vi "Restart.CheckValidSelection.vi"(8 "error in (no error)":errorcluster, 10 "Restart Path":path, 11 "State Variables":T1={"Events.State"=refnum, "Events.Test Result"=refnum, "Events.Progress"=refnum, "INI.Settings"={"Build Location"=path "C:/Simple Sequence Editor/SequenceRepo", "LoggingLocation"=path "", "Sequence.AbortChannel"="", "Sequence.IterationInfoChannel"="", "Sequence.DurationChannel"="", "Sequence.StepInfoChannel"="", "Sequence.SkipChannel"="", "PlotChannels"=[], "Sequence.InitializeScript"=path "C:/Simple Sequence Editor/SequenceRepo", "Sequence.CleanupScript"=path "", "Log.DefaultRate"=0.0}, "NIVS.AlarmManager"=refnum, "NIVS.BaseLogPath"=path "", "NIVS.DataLogManagerRef"=refnum, "NIVS.DataLogSpecRef"=refnum, "NIVS.Deployed"=FALSE, "NIVS.Events"={"SequenceEvent"=refnum, "SystemChangeEvent"=refnum, "WorkspaceEvent"=refnum}, "NIVS.GatewayIPAddress"="", "NIVS.DataLogGUID"="", "NIVS.ProfileCallback"=refnum, "NIVS.ProfileRef"=refnum, "NIVS.SequenceState"=enum."Idle", "NIVS.SystemDefinitionFile"=path "", "NIVS.SystemStateRefs"={"CustDatRef"=refnum, "EvtRef"=refnum, "Target State User Event"=refnum}, "NIVS.WorkspaceManager"=refnum, "NIVS.EventLogGUID"="", "NIVS.EventLogManagerRef"=refnum, "NIVS.EventLogSpecRef"=refnum, "NIVS.BaseToolPath"=path "", "Restart.Path"=path "", "Sequence.#ofColumns"=0, "Sequence.Iterations"=0, "Sequence.Channels"=[], "Sequence.ValidConfig?"=FALSE, "Station.ID"="", "UDP.Queue"=refnum, "UI.Abort"=refnum, "UI.Alarms"=refnum, "UI.Apply"=refnum, "UI.Back"=refnum, "UI.BaseFileName"=refnum, "UI.CurrentIteration"=refnum, "UI.CurrentStep"=refnum, "UI.CyclicFrequency"=refnum, "UI.Description"=refnum, "UI.DelayTime"=refnum, "UI.DisableAlarms"=refnum, "UI.Duration"=refnum, "UI.EnableLogging"=refnum, "UI.EnableState"=refnum, "UI.High"=refnum, "UI.LogChannels"=refnum, "UI.Low"=refnum, "UI.MonitoredVariable"=refnum, "UI.Next"=refnum, "UI.NumberOfCycles"=refnum, "UI.OperatorName"=refnum, "UI.Pause"=refnum, "UI.Profile"=refnum, "UI.Revert"=refnum, "UI.Skip"=refnum, "UI.Start"=refnum, "UI.StartIteration"=refnum, "UI.StartStep"=refnum, "UI.TabControl"=refnum, "UI.TotalIterations"=refnum, "UI.WaveformDefinition"=refnum, "UI.WaveformPreview"=refnum, "UI.WorkOrderNumber"=refnum, "UI.Chart"=refnum, "UI.Status"=refnum, "UI.DataView"=refnum, "UI.Table"=refnum, "UI.Multihead"=refnum, "UI.ToolTab"=refnum, "UI.Result"=refnum, "UI.Log Path"=refnum, "UI.ReportPath"=refnum, "UI.RestartPath"=refnum, "UI.AlarmLog"=refnum}) -> (0 "error out":errorcluster, 2 "Load Restart?":bool, 3 "State Variables out":T1={"Events.State"=refnum, "Events.Test Result"=refnum, "Events.Progress"=refnum, "INI.Settings"={"Build Location"=path "C:/Simple Sequence Editor/SequenceRepo", "LoggingLocation"=path "", "Sequence.AbortChannel"="", "Sequence.IterationInfoChannel"="", "Sequence.DurationChannel"="", "Sequence.StepInfoChannel"="", "Sequence.SkipChannel"="", "PlotChannels"=[], "Sequence.InitializeScript"=path "C:/Simple Sequence Editor/SequenceRepo", "Sequence.CleanupScript"=path "", "Log.DefaultRate"=0.0}, "NIVS.AlarmManager"=refnum, "NIVS.BaseLogPath"=path "", "NIVS.DataLogManagerRef"=refnum, "NIVS.DataLogSpecRef"=refnum, "NIVS.Deployed"=FALSE, "NIVS.Events"={"SequenceEvent"=refnum, "SystemChangeEvent"=refnum, "WorkspaceEvent"=refnum}, "NIVS.GatewayIPAddress"="", "NIVS.DataLogGUID"="", "NIVS.ProfileCallback"=refnum, "NIVS.ProfileRef"=refnum, "NIVS.SequenceState"=enum."Idle", "NIVS.SystemDefinitionFile"=path "", "NIVS.SystemStateRefs"={"CustDatRef"=refnum, "EvtRef"=refnum, "Target State User Event"=refnum}, "NIVS.WorkspaceManager"=refnum, "NIVS.EventLogGUID"="", "NIVS.EventLogManagerRef"=refnum, "NIVS.EventLogSpecRef"=refnum, "NIVS.BaseToolPath"=path "", "Restart.Path"=path "", "Sequence.#ofColumns"=0, "Sequence.Iterations"=0, "Sequence.Channels"=[], "Sequence.ValidConfig?"=FALSE, "Station.ID"="", "UDP.Queue"=refnum, "UI.Abort"=refnum, "UI.Alarms"=refnum, "UI.Apply"=refnum, "UI.Back"=refnum, "UI.BaseFileName"=refnum, "UI.CurrentIteration"=refnum, "UI.CurrentStep"=refnum, "UI.CyclicFrequency"=refnum, "UI.Description"=refnum, "UI.DelayTime"=refnum, "UI.DisableAlarms"=refnum, "UI.Duration"=refnum, "UI.EnableLogging"=refnum, "UI.EnableState"=refnum, "UI.High"=refnum, "UI.LogChannels"=refnum, "UI.Low"=refnum, "UI.MonitoredVariable"=refnum, "UI.Next"=refnum, "UI.NumberOfCycles"=refnum, "UI.OperatorName"=refnum, "UI.Pause"=refnum, "UI.Profile"=refnum, "UI.Revert"=refnum, "UI.Skip"=refnum, "UI.Start"=refnum, "UI.StartIteration"=refnum, "UI.StartStep"=refnum, "UI.TabControl"=refnum, "UI.TotalIterations"=refnum, "UI.WaveformDefinition"=refnum, "UI.WaveformPreview"=refnum, "UI.WorkOrderNumber"=refnum, "UI.Chart"=refnum, "UI.Status"=refnum, "UI.DataView"=refnum, "UI.Table"=refnum, "UI.Multihead"=refnum, "UI.ToolTab"=refnum, "UI.Result"=refnum, "UI.Log Path"=refnum, "UI.ReportPath"=refnum, "UI.RestartPath"=refnum, "UI.AlarmLog"=refnum})   [LabVIEW 2015, in "Single Station Execution.lvlib"]
uses:
  Single Station Execution.lvlib
  <vilib>/NI Veristand/Execution/Workspace/SystemStateEventRef.ctl
  <vilib>/NI Veristand/Execution/Workspace/NI_VS Workspace ExecutionAPI.lvlib
  NationalInstruments.VeriStand.ClientAPI
  <vilib>/NI Veristand/Execution/Workspace/WorkspaceAPI.ctl
  Types/Execution.SequenceState.ctl
  <vilib>/NI Veristand/Execution/DataLogging/DataLoggingSpecification Ref.ctl
  <vilib>/NI Veristand/Execution/DataLogging/NI_VS Data Logging API.lvlib
  <vilib>/NI Veristand/Execution/DataLogging/IDataLogging Ref.ctl
  <vilib>/NI Veristand/Execution/Workspace/SystemStateRegEventRef.ctl
  Types/Execute.UserEventRefs.ctl
  Types/Main.StateVariables.ctl
  <vilib>/NI Veristand/Execution/Workspace/Target State.ctl
  <vilib>/NI Veristand/Execution/Workspace/Target State Info.ctl
  NationalInstruments.VeriStand.RealTimeSequenceDefinitionApi
  <vilib>/NI Veristand/Execution/AlarmManager/AlarmManagerAPI.ctl
  <vilib>/NI Veristand/Execution/AlarmManager/NI_VS AlarmManager ExecutionAPI.lvlib
  Types/INI.Settings.ctl
  Types/UDPEngine.State.ctl
  Types/UDPEngine.QueueCluster.ctl
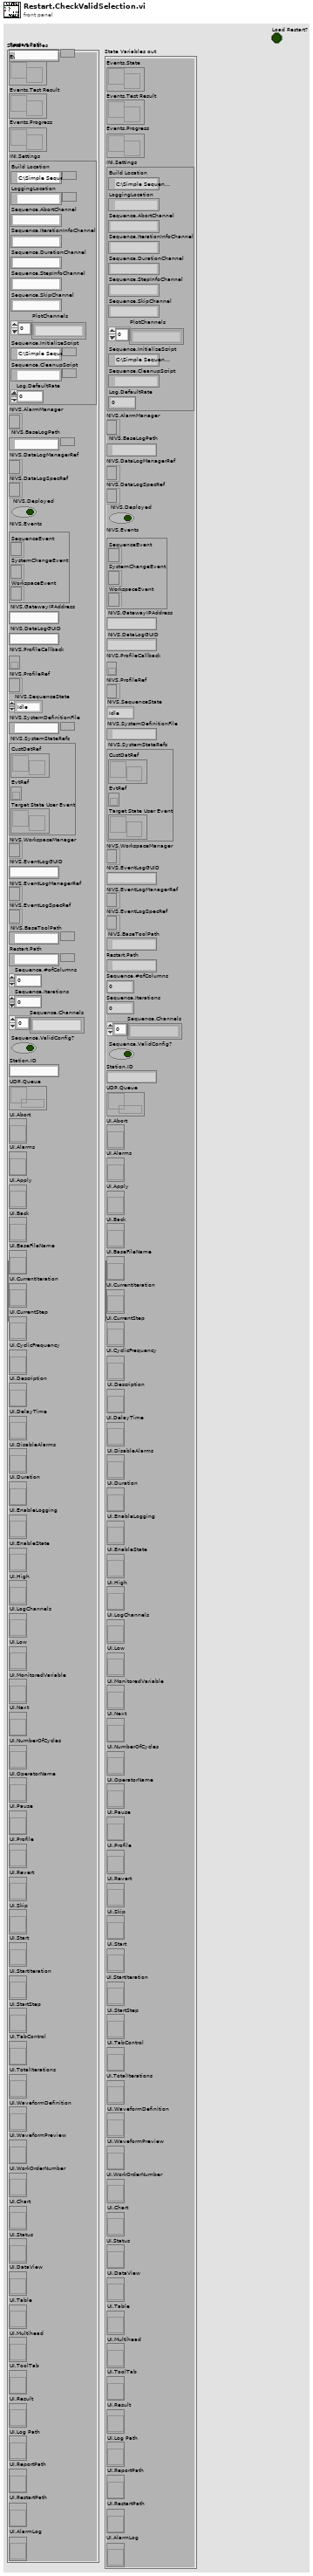
[diagram p1: front panel]
types:
  T1 = typedef "Single Station Execution.lvlib/Main.StateVariables.ctl" = cluster{"Events.State":refnum<user-event>, "Events.Test Result":refnum<user-event>, "Events.Progress":refnum<user-event>, "INI.Settings":T2, "NIVS.AlarmManager":T3, "NIVS.BaseLogPath":path, "NIVS.DataLogManagerRef":T4, "NIVS.DataLogSpecRef":T5, "NIVS.Deployed":bool, "NIVS.Events":T6, "NIVS.GatewayIPAddress":string, "NIVS.DataLogGUID":string, "NIVS.ProfileCallback":refnum<k27>, "NIVS.ProfileRef":refnum<k24>, "NIVS.SequenceState":T8, "NIVS.SystemDefinitionFile":path, "NIVS.SystemStateRefs":T9, "NIVS.WorkspaceManager":T10, "NIVS.EventLogGUID":string, "NIVS.EventLogManagerRef":T4, "NIVS.EventLogSpecRef":T5, "NIVS.BaseToolPath":path, "Restart.Path":path, "Sequence.#ofColumns":i32, "Sequence.Iterations":u32, "Sequence.Channels":string[], "Sequence.ValidConfig?":bool, "Station.ID":string, "UDP.Queue":refnum<queue>, "UI.Abort":refnum<vi>, "UI.Alarms":refnum<vi>, "UI.Apply":refnum<vi>, "UI.Back":refnum<vi>, "UI.BaseFileName":refnum<vi>, "UI.CurrentIteration":refnum<vi>, "UI.CurrentStep":refnum<vi>, "UI.CyclicFrequency":refnum<vi>, "UI.Description":refnum<vi>, "UI.DelayTime":refnum<vi>, "UI.DisableAlarms":refnum<vi>, "UI.Duration":refnum<vi>, "UI.EnableLogging":refnum<vi>, "UI.EnableState":refnum<vi>, "UI.High":refnum<vi>, "UI.LogChannels":refnum<vi>, "UI.Low":refnum<vi>, "UI.MonitoredVariable":refnum<vi>, "UI.Next":refnum<vi>, "UI.NumberOfCycles":refnum<vi>, "UI.OperatorName":refnum<vi>, "UI.Pause":refnum<vi>, "UI.Profile":refnum<vi>, "UI.Revert":refnum<vi>, "UI.Skip":refnum<vi>, "UI.Start":refnum<vi>, "UI.StartIteration":refnum<vi>, "UI.StartStep":refnum<vi>, "UI.TabControl":refnum<vi>, "UI.TotalIterations":refnum<vi>, "UI.WaveformDefinition":refnum<vi>, "UI.WaveformPreview":refnum<vi>, "UI.WorkOrderNumber":refnum<vi>, "UI.Chart":refnum<vi>, "UI.Status":refnum<vi>, "UI.DataView":refnum<vi>, "UI.Table":refnum<vi>, "UI.Multihead":refnum<vi>, "UI.ToolTab":refnum<vi>, "UI.Result":refnum<vi>, "UI.Log Path":refnum<vi>, "UI.ReportPath":refnum<vi>, "UI.RestartPath":refnum<vi>, "UI.AlarmLog":refnum<vi>}
  T2 = typedef "Single Station Execution.lvlib/INI.Settings.ctl" = cluster{"Build Location":path, "LoggingLocation":path, "Sequence.AbortChannel":string, "Sequence.IterationInfoChannel":string, "Sequence.DurationChannel":string, "Sequence.StepInfoChannel":string, "Sequence.SkipChannel":string, "PlotChannels":string[], "Sequence.InitializeScript":path, "Sequence.CleanupScript":path, "Log.DefaultRate":dbl}
  T3 = typedef "NI_VS AlarmManager ExecutionAPI.lvlib/AlarmManagerAPI.ctl" = refnum<k24>
  T4 = typedef "NI_VS Data Logging API.lvlib/IDataLogging Ref.ctl" = refnum<k24>
  T5 = typedef "NI_VS Data Logging API.lvlib/DataLoggingSpecification Ref.ctl" = refnum<k24>
  T6 = typedef "Single Station Execution.lvlib/Execute.UserEventRefs.ctl" = cluster{"SequenceEvent":refnum<event-registration>, "SystemChangeEvent":T7, "WorkspaceEvent":refnum<event-registration>}
  T7 = typedef "NI_VS Workspace ExecutionAPI.lvlib/SystemStateRegEventRef.ctl" = refnum<event-registration>
  T8 = typedef "Single Station Execution.lvlib/Execution.SequenceState.ctl" = enum16{"Idle", "Initializing", "Running", "Paused", "Finalizing", "Complete"}
  T9 = typedef "NI_VS Workspace ExecutionAPI.lvlib/SystemStateEventRef.ctl" = cluster{"CustDatRef":refnum<user-event>, "EvtRef":refnum<k27>, "Target State User Event":refnum<user-event>}
  T10 = typedef "NI_VS Workspace ExecutionAPI.lvlib/WorkspaceAPI.ctl" = refnum<k24>
  T11 = typedef "Single Station Execution.lvlib/Restart.Settings.ctl" = cluster{"LogFile":path, "Log Settings":T12[], "StimulusProfile":path, "StopIteration":u32, "StopStep":u32, "Log Channels":T16, "Base File Name":string, "Enable Logging":bool, "Profile":string, "StopDuration":dbl, "Waveform Definition":path, "Number of Cycles":dbl, "Cyclic Frequency":dbl, "Work Order Number":string, "Operator Name":string, "Description":string, "Station.ID":string, "Sequence.Channels":string[], "Alarms":T17[]}
  T12 = typedef "NI_VS Data Logging API.lvlib/TDMS Channel Group.ctl" = cluster{"Group Name":string, "Group Description":string, "Group Properties":T13[], "Channels":T14[], "Time Channel Options":T15, "Time Channel Name":string}
  T13 = typedef "NI_VS Data Logging API.lvlib/TDMS Property.ctl" = cluster{"Name":string, "Value":variant}
  T14 = typedef "NI_VS Data Logging API.lvlib/TDMS Channel.ctl" = cluster{"Channel Name":string, "Channel Path":string, "Channel Description":string, "Channel Properties":T13[]}
  T15 = typedef "NI_VS Data Logging API.lvlib/Time Channel Options.ctl" = enum16{"No Time Channel", "Absolute Time", "System Time", "System Time - Microseconds", "Absolute Time as Double", "Relative To First Start Trigger", "Relative To Session Start"}
  T16 = typedef "Single Station Execution.lvlib/Log.SelectedChannels.ctl" = enum16{"Channels (No System Channel)", "Aliases", "All"}
  T17 = typedef "Single Station Execution.lvlib/Config.AlarmSettings.ctl" = cluster{"Watch Channel":string, "High Limit":dbl, "Low Limit":dbl, "Delay":dbl, "State":enum16{"Disabled", "Enabled", "Tripped", "Delayed Trip", "Indicate"}, "Alarm Name":string}
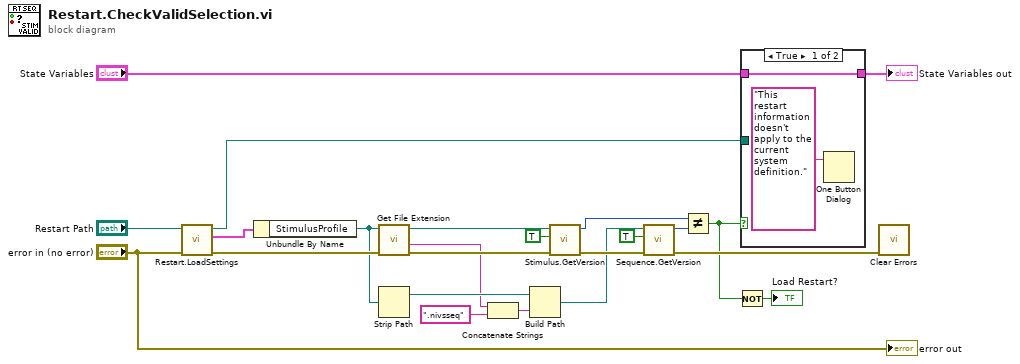
[diagram p0: block diagram]
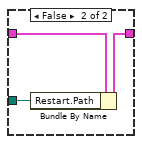
[diagram p2: hidden frame]
diagram:
  n1 = call "Restart.LoadSettings.vi"("error in"="error in (no error)", "path (use dialog)"="Restart Path") -> ("error out"=w8:errorcluster, "Restart Settings"=w22:T11, "path"=w21:path)  [unwired: 7 in]
  n2 = Unbundle By Name(w22) -> ("StimulusProfile"=w5:path)
  n3 = call <vilib>:"Get File Extension.vi"("error in (no error)"=w8, "file"=w5) -> ("error out"=w7:errorcluster, "filename without extension"=w3:string, "dup file"=w6:path)  [unwired: 5 in, 2 out]
  n4 = Strip Path(path=w5) -> (stripped path=w4:path)  [unwired: 1 out]
  n5 = Concatenate Strings(w3, ".nivsseq" ("string")) -> (w2:string)
  n6 = Build Path(base path=w4, name or relative path=w2) -> (appended path=w14:path)
  n7 = call "Stimulus.GetVersion.vi"("error in (no error)"=w7, "Exists"=TRUE, "Path"=w6) -> ("error out"=w17:errorcluster, "Build"=w15:u32)  [unwired: 7 in]
  n8 = call "Sequence.GetVersion.vi"("error in (no error)"=w17, "Exists"=TRUE, "Path"=w14) -> ("error out"=w13:errorcluster, "Build"=w16:u32)  [unwired: 7 in]
  n9 = Not Equal?(x=w15, y=w16) -> (x != y?=w9:bool)
  n10 = Not(x=w9) -> (.not. x?=→"Load Restart?":bool)
  n11 = case shown="True" w9 {
    tunnel: [w25 w28] -> w19
    tunnel: w21 -> [_ w27]
    tunnel: "State Variables" -> [w25 w26]
    frame True {
      n12 = One Button Dialog(message="This restart information doesn't apply to the current system definition.") -> ()  [unwired: 1 in, 1 out]
    }
    frame False {
      n13 = Bundle By Name(cluster=w26, "Restart.Path"=w27) -> (w28:T1)
    }
  }
  "State Variables out" <- w19
  n14 = call <vilib>:"Clear Errors.vi"("error in (no error)"=w13) -> ()  [unwired: 5 in, 2 out]
  "error out" <- "error in (no error)"
